vi "DIO_Close.vi"(0 "output cluster 3":T1) -> ()   [LabVIEW 2015]
uses:
  Periodic Task/Ref_Num/DIO_Type_Def.ctl
  <vilib>/Rock Robotics/WPI/Ultrasonic/WPI_SonarMB1010DigitalDeviceRef.ctl
  <vilib>/Rock Robotics/WPI/Counter/WPI_CounterDevRef.ctl
  <vilib>/Rock Robotics/SystemInterfaces/Counter/FPGA_CounterCtrSystemIndex.ctl
  <vilib>/Rock Robotics/WPI/Encoder/WPI_EncoderDevRef.ctl
  <vilib>/Rock Robotics/SystemInterfaces/Encoder/FPGA_EncoderIdx.ctl
  <vilib>/Rock Robotics/WPI/Encoder/WPI_EncoderType.ctl
  <vilib>/Rock Robotics/WPI/DigitalInput/WPI_DigitalInputDevRef.ctl
  <vilib>/Rock Robotics/SystemInterfaces/DIO/FPGA_DIOChannel.ctl
  <vilib>/Rock Robotics/WPI/Ultrasonic/WPI_SonarMB1010DigitalClose.vi
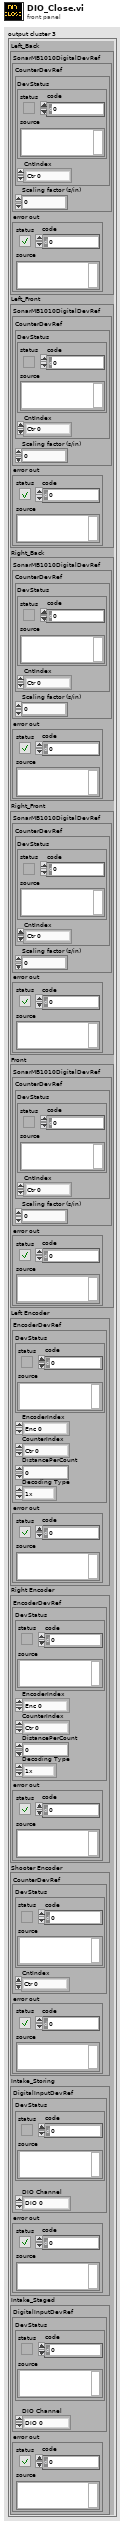
[diagram p1: front panel]
types:
  T1 = typedef "DIO_Type_Def.ctl" = cluster{"Left_Back":cluster{"SonarMB1010DigitalDevRef":T2, "error out":errorcluster}, "Left_Front":cluster{"SonarMB1010DigitalDevRef":T2, "error out":errorcluster}, "Right_Back":cluster{"SonarMB1010DigitalDevRef":T2, "error out":errorcluster}, "Right_Front":cluster{"SonarMB1010DigitalDevRef":T2, "error out":errorcluster}, "Front":cluster{"SonarMB1010DigitalDevRef":T2, "error out":errorcluster}, "Left Encoder":cluster{"EncoderDevRef":T5, "error out":errorcluster}, "Right Encoder":cluster{"EncoderDevRef":T5, "error out":errorcluster}, "Shooter Encoder":cluster{"CounterDevRef":T3, "error out":errorcluster}, "Intake_Storing":cluster{"DigitalInputDevRef":T8, "error out":errorcluster}, "Intake_Staged":cluster{"DigitalInputDevRef":T8, "error out":errorcluster}}
  T2 = typedef "WPI_SonarMB1010DigitalDeviceRef.ctl" = cluster{"CounterDevRef":T3, "Scaling factor (s/in)":dbl}
  T3 = typedef "WPI_CounterDevRef.ctl" = cluster{"DevStatus":errorcluster, "CntIndex":T4}
  T4 = typedef "FPGA_CounterCtrSystemIndex.ctl" = enum8{"Ctr 0", "Ctr 1", "Ctr 2", "Ctr 3", "Ctr 4", "Ctr 5", "Ctr 6", "Ctr 7", "Invalid"}
  T5 = typedef "WPI_EncoderDevRef.ctl" = cluster{"DevStatus":errorcluster, "EncoderIndex":T6, "CounterIndex":T4, "DistancePerCount":dbl, "Decoding Type":T7}
  T6 = typedef "FPGA_EncoderIdx.ctl" = enum8{"Enc 0", "Enc 1", "Enc 2", "Enc 3", "Enc 4", "Enc 5", "Enc 6", "Enc 7", "Invalid"}
  T7 = typedef "WPI_EncoderType.ctl" = enum16{"1x", "2x", "4x"}
  T8 = typedef "WPI_DigitalInputDevRef.ctl" = cluster{"DevStatus":errorcluster, "DIO Channel":T9}
  T9 = typedef "FPGA_DIOChannel.ctl" = enum8{"DIO 0", "DIO 1", "DIO 2", "DIO 3", "DIO 4", "DIO 5", "DIO 6", "DIO 7", "DIO 8", "DIO 9", "DIO MXP 0", "DIO MXP 1", "DIO MXP 2", "DIO MXP 3", "DIO MXP 4", "DIO MXP 5", "DIO MXP 6", "DIO MXP 7", "DIO MXP 8", "DIO MXP 9", "DIO MXP 10", "DIO MXP 11", "DIO MXP 12", "DIO MXP 13", "DIO MXP 14", "DIO MXP 15", "Invalid"}
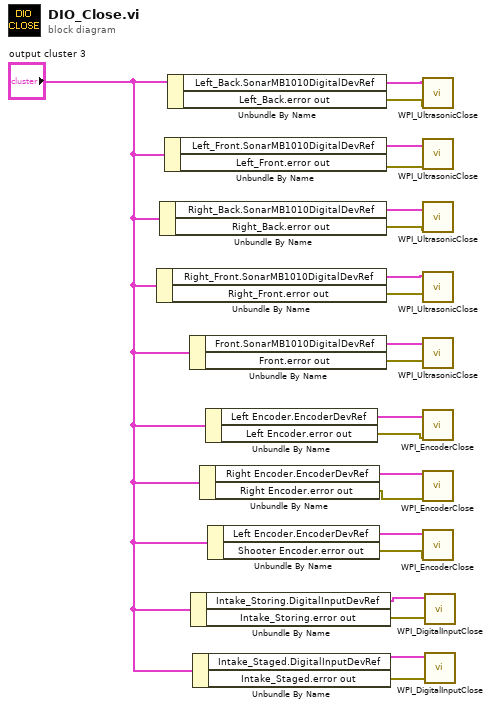
[diagram p0: block diagram]
diagram:
  n1 = Unbundle By Name("output cluster 3") -> ("Right_Front.SonarMB1010DigitalDevRef"=w15:T2, "Right_Front.error out"=w14:errorcluster)
  n2 = Unbundle By Name("output cluster 3") -> ("Right_Back.SonarMB1010DigitalDevRef"=w17:T2, "Right_Back.error out"=w16:errorcluster)
  n3 = Unbundle By Name("output cluster 3") -> ("Left_Front.SonarMB1010DigitalDevRef"=w19:T2, "Left_Front.error out"=w18:errorcluster)
  n4 = Unbundle By Name("output cluster 3") -> ("Left_Back.SonarMB1010DigitalDevRef"=w21:T2, "Left_Back.error out"=w20:errorcluster)
  n5 = Unbundle By Name("output cluster 3") -> ("Front.SonarMB1010DigitalDevRef"=w13:T2, "Front.error out"=w12:errorcluster)
  n6 = Unbundle By Name("output cluster 3") -> ("Intake_Storing.DigitalInputDevRef"=w5:T8, "Intake_Storing.error out"=w4:errorcluster)
  n7 = Unbundle By Name("output cluster 3") -> ("Intake_Staged.DigitalInputDevRef"=w3:T8, "Intake_Staged.error out"=w2:errorcluster)
  n8 = Unbundle By Name("output cluster 3") -> ("Right Encoder.EncoderDevRef"=w9:T5, "Right Encoder.error out"=w8:errorcluster)
  n9 = Unbundle By Name("output cluster 3") -> ("Left Encoder.EncoderDevRef"=w11:T5, "Left Encoder.error out"=w10:errorcluster)
  n10 = Unbundle By Name("output cluster 3") -> ("Left Encoder.EncoderDevRef"=w7:T5, "Shooter Encoder.error out"=w6:errorcluster)
  n11 = call-poly <vilib>:"WPI_UltrasonicClose.vi"("error in (no error)"=w20, "SonarMB1010DigitalDevRef"=w21) -> ()  [unwired: 9 in, 1 out]
  n12 = call-poly <vilib>:"WPI_UltrasonicClose.vi"("error in (no error)"=w18, "SonarMB1010DigitalDevRef"=w19) -> ()  [unwired: 9 in, 1 out]
  n13 = call-poly <vilib>:"WPI_UltrasonicClose.vi"("error in (no error)"=w16, "SonarMB1010DigitalDevRef"=w17) -> ()  [unwired: 9 in, 1 out]
  n14 = call-poly <vilib>:"WPI_UltrasonicClose.vi"("error in (no error)"=w14, "SonarMB1010DigitalDevRef"=w15) -> ()  [unwired: 9 in, 1 out]
  n15 = call-poly <vilib>:"WPI_UltrasonicClose.vi"("error in (no error)"=w12, "SonarMB1010DigitalDevRef"=w13) -> ()  [unwired: 9 in, 1 out]
  n16 = call <vilib>:"WPI_EncoderClose.vi"("error in (no error)"=w10, "EncoderDevRef"=w11) -> ()  [unwired: 9 in, 1 out]
  n17 = call <vilib>:"WPI_EncoderClose.vi"("error in (no error)"=w8, "EncoderDevRef"=w9) -> ()  [unwired: 9 in, 1 out]
  n18 = call <vilib>:"WPI_EncoderClose.vi"("error in (no error)"=w6, "EncoderDevRef"=w7) -> ()  [unwired: 9 in, 1 out]
  n19 = call <vilib>:"WPI_DigitalInputClose.vi"("error in (no error)"=w4, "DigitalInputDevRef"=w5) -> ()  [unwired: 9 in, 1 out]
  n20 = call <vilib>:"WPI_DigitalInputClose.vi"("error in (no error)"=w2, "DigitalInputDevRef"=w3) -> ()  [unwired: 9 in, 1 out]
